vi "obstacle avoidance.vi"(11 "allowed proximity squared":i16=400) -> ()   [LabVIEW 2010]
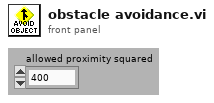
[diagram p1: front panel]
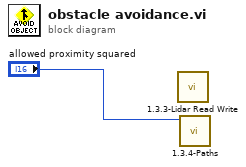
[diagram p0: block diagram]
diagram:
  n1 = call "1.3.3-Lidar Read Write.vi"() -> ()  [unwired: 1 in]
  n2 = call "1.3.4-Paths.vi"("allowed proximity squared"="allowed proximity squared") -> ()  [unwired: 11 in]
